vi "TakeData.vi"(8 "error in":errorcluster, 9 "#words":u32, 10 "Location":u32, 11 "Port":refnum<visa-resource-name>) -> (0 "error out":errorcluster, 1 "read buffer":string, 2 "Data":u16[](array[numeric]) format="%04x", 3 "Port out":refnum<visa-resource-name>)   [LabVIEW 2021]
uses:
  5c735bce-767e-4a53-8910-193faff062d0.vi
panel:
  out "Data 2":u16[](array[numeric]) format="%04x"
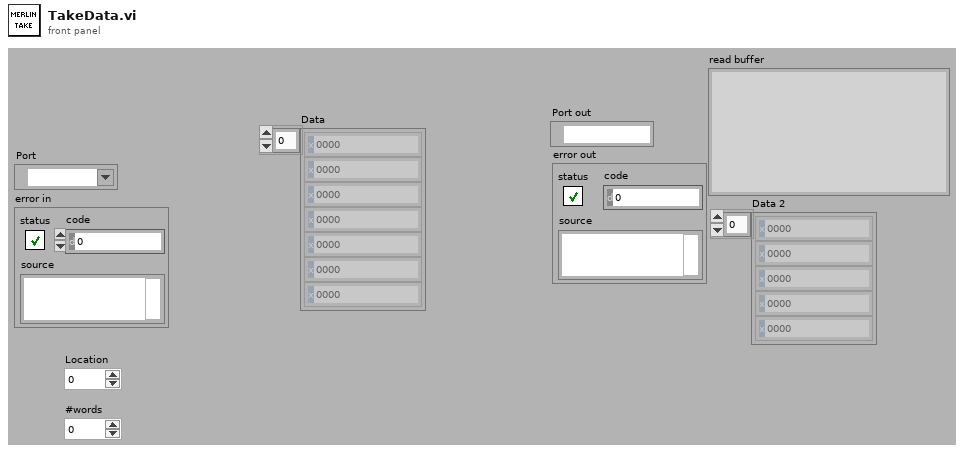
[diagram p1: front panel]
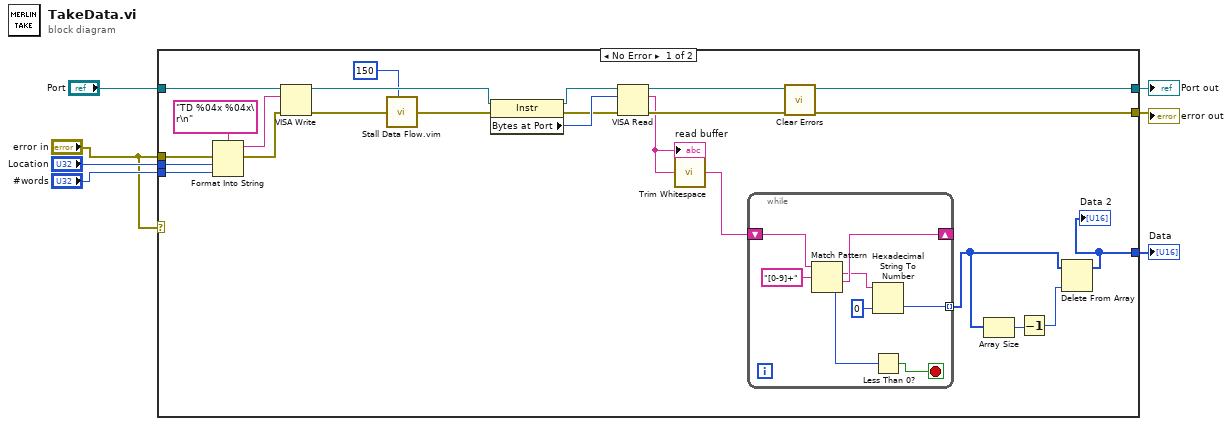
[diagram p0: block diagram]
diagram:
  n1 = case shown="No Error" "error in" {
    selector: "error in" -> [_ w39]
    tunnel: "Port" -> [w28 w40]
    tunnel: [w27 w40] -> w6
    tunnel: "error in" -> [w25 _]
    tunnel: [w23 w39] -> w5
    tunnel: "Location" -> [w22 _]
    tunnel: "#words" -> [w21 _]
    tunnel: [w15 _] -> w2
    frame No Error {
      n2 = Format Into String(format string="TD %04x %04x\r\n" ("concatenated string"), error in=w25, w22, w21) -> (resulting string=w29:string, error out=w26:errorcluster)  [unwired: 1 in]
      n3 = VISA Write(VISA resource name=w28, write buffer=w29, error in (no error)=w26) -> (VISA resource name out=w14:refnum<visa-resource-name>, error out=w11:errorcluster)  [unwired: 1 out]
      n4 = call "Stall Data Flow.vim"("value in"=w11, "milliseconds to wait"=u32 150) -> ("value out"=w9:errorcluster)  [unwired: 1 out]
      n5 = property class="Instr"(reference=w14, error in=w9) -> (reference out=w13:refnum<visa-resource-name>, error out=w10:errorcluster, "Bytes at Port"=w12:u32)
      n6 = VISA Read(VISA resource name=w13, byte count=w12, error in (no error)=w10) -> (VISA resource name out=w27:refnum<visa-resource-name>, read buffer=w20:string, error out=w24:errorcluster)  [unwired: 1 out]
      "read buffer" <- w20
      n7 = call <vilib>:"Trim Whitespace.vi"("string"=w20) -> ("trimmed string"=w19:string)  [unwired: 1 in]
      n8 = while {
        shift-right: [w36] -> _
        shift-left: w19 -> [w38]
        tunnel: [w33] -> w18 mode=indexing
        stop <- w31 stop-if-true
        n9 = Match Pattern(string=w38, regular expression="[0-9]+") -> (match substring=w35:string, after substring=w36:string, offset past match=w32:i32)  [unwired: 1 in, 1 out]
        n10 = Hexadecimal String To Number(string=w35, default (0uL)=u16 0 ("default (0 U32)")) -> (number=w33:u16)  [unwired: 1 in, 1 out]
        n11 = Less Than 0?(x=w32) -> (x < 0?=w31:bool)
      }
      n12 = call <vilib>:"Clear Errors.vi"("error in (no error)"=w24) -> ("error out"=w23:errorcluster)  [unwired: 5 in, 1 out]
      n13 = Array Size(array=w18) -> (size(s)=w17:i32)
      n14 = Decrement(x=w17) -> (x-1=w16:i32)
      n15 = Delete From Array(array=w18, index=w16) -> (array with subset deleted=w15:u16[])  [unwired: 1 in, 1 out]
      "Data 2" <- w15
    }
    frame Error {
    }
  }
  "Port out" <- w6
  "error out" <- w5
  "Data" <- w2
